vi "Sounds.vi"(8 "error in":errorcluster, 11 "choice in":enum16{"Victory", "GameOver"}(ring)) -> (0 "error out":errorcluster)   [LabVIEW 2010, in "Labricks.lvlib" / "Game.lvclass"]
uses:
  Game.lvclass
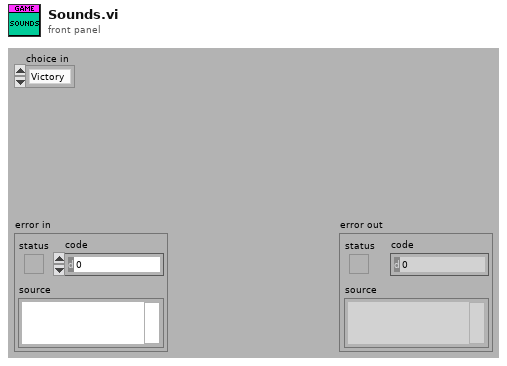
[diagram p1: front panel]
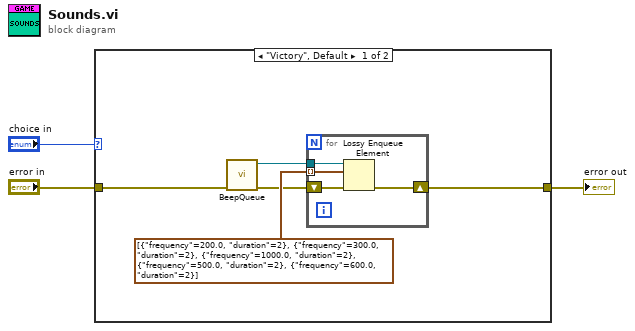
[diagram p0: block diagram]
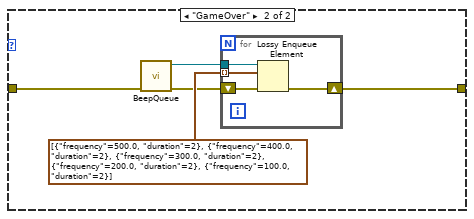
[diagram p2: hidden frame]
diagram:
  n1 = case shown="\"Victory\", Default" "choice in" {
    tunnel: "error in" -> [w5 w14]
    tunnel: [w4 w13] -> w2
    frame "Victory", Default {
      n2 = call "BeepQueue.vi"("error in"=w5) -> ("error out"=w7:errorcluster, "queue out"=w6:refnum<queue>)  [unwired: 5 in]
      n3 = for {
        tunnel: w6 -> [w12]
        tunnel: cluster{"frequency":dbl, "duration":i32}[] [{"frequency"=200.0, "duration"=2}, {"frequency"=300.0, "duration"=2}, {"frequency"=1000.0, "duration"=2}, {"frequency"=500.0, "duration"=2}, {"frequency"=600.0, "duration"=2}] -> [w9] mode=indexing
        shift-right: [w10] -> w4
        shift-left: w7 -> [w11]
        n4 = Lossy Enqueue Element(queue=w12, element=w9, error in (no error)=w11) -> (error out=w10:errorcluster)  [unwired: 3 out]
      }
    }
    frame "GameOver" {
      n5 = call "BeepQueue.vi"("error in"=w14) -> ("error out"=w16:errorcluster, "queue out"=w15:refnum<queue>)  [unwired: 5 in]
      n6 = for {
        tunnel: w15 -> [w21]
        tunnel: cluster{"frequency":dbl, "duration":i32}[] [{"frequency"=500.0, "duration"=2}, {"frequency"=400.0, "duration"=2}, {"frequency"=300.0, "duration"=2}, {"frequency"=200.0, "duration"=2}, {"frequency"=100.0, "duration"=2}] -> [w18] mode=indexing
        shift-right: [w19] -> w13
        shift-left: w16 -> [w20]
        n7 = Lossy Enqueue Element(queue=w21, element=w18, error in (no error)=w20) -> (error out=w19:errorcluster)  [unwired: 3 out]
      }
    }
  }
  "error out" <- w2
